vi "Write Settings.vi"(8 "error in":errorcluster, 10 "Settings":T1, 11 "PowerSupply in":refnum<class "PowerSupply.lvclass">) -> (0 "error out":errorcluster, 3 "PowerSupply out":refnum<class "PowerSupply.lvclass">)   [LabVIEW 2019, in "PowerSupply.lvlib" / "PowerSupply.lvclass"]
uses:
  Library/PowerSupply.lvclass
  Custom Controls/Settings.ctl
  Custom Controls/OCP Mode.ctl
  Custom Controls/Sense Point.ctl
  Library/PowerSupply.lvclass/PowerSupply.ctl
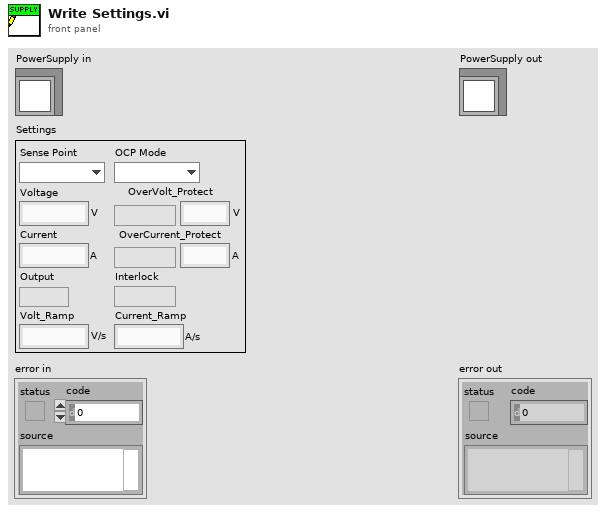
[diagram p1: front panel]
types:
  T1 = typedef "PowerSupply.lvlib/PowerSupply.lvclass/Settings.ctl" = cluster{"Volt_Ramp":dbl, "Output":bool, "Current":dbl, "Voltage":dbl, "Current_Ramp":dbl, "Interlock":bool, "OCP":bool, "OverCurrent_Protect":dbl, "OVP":bool, "OverVolt_Protect":dbl, "OCP Mode":T2, "Sense Point":T3}
  T2 = typedef "PowerSupply.lvlib/PowerSupply.lvclass/OCP Mode.ctl" = enum16{"Shutdown", "Foldback"}
  T3 = typedef "PowerSupply.lvlib/PowerSupply.lvclass/Sense Point.ctl" = enum16{"Local", "Remote"}
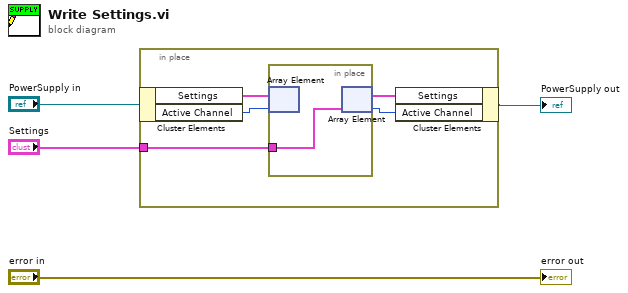
[diagram p0: block diagram]
diagram:
  n1 = in-place {
    in-place-border: "Settings" -> [w5]
    n2 = in-place-cluster #1("PowerSupply in") -> ("Settings"=w9:T1[], "Active Channel"=w8:u32)
    n3 = in-place {
      in-place-border: w5 -> [w10]
      n4 = in-place-array #2(w9, w8) -> ()  [unwired: 1 out]
      n5 = in-place-array #2(w10) -> (w7:T1[], w6:i32)
    }
    n6 = in-place-cluster #1("Settings"=w7, "Active Channel"=w6) -> (→"PowerSupply out":refnum<class "PowerSupply.lvclass">)
  }
  "error out" <- "error in"
